vi "Calculate Distance to Target.vi"(10 "Diff Top X to Bottom X":dbl, 11 "Camera Height (pix)":dbl=320.0) -> (1 "Distance to Wall (in.)":dbl)   [LabVIEW 2019]
panel:
  in  "Camera Pix Hight Angle (degrees)":dbl=19.0
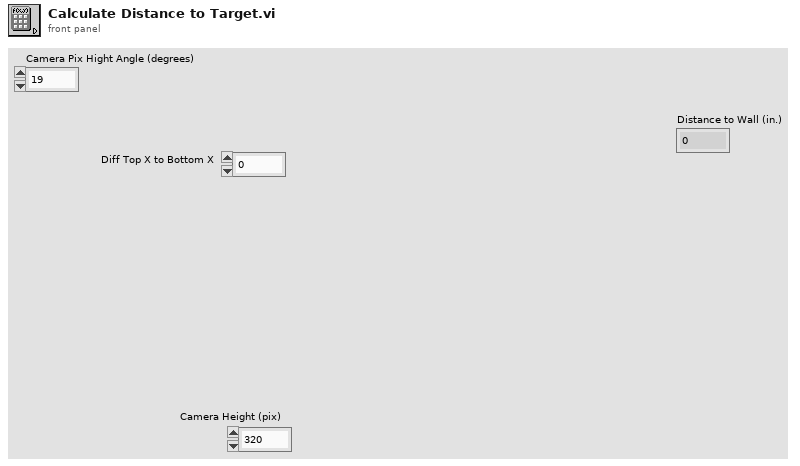
[diagram p1: front panel]
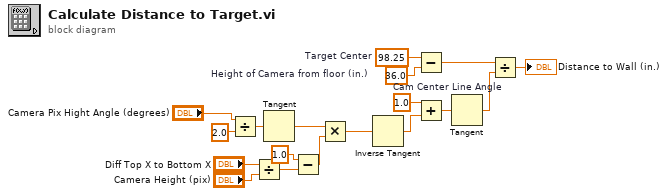
[diagram p0: block diagram]
diagram:
  w2 = 1.0  # Cam Center Line Angle
  w17 = 36.0  # Height of Camera from floor (in.)
  w18 = 98.25  # Target Center
  n1 = Divide(x="Camera Pix Hight Angle (degrees)", y=2.0) -> (x/y=w14:dbl)
  n2 = Divide(x="Diff Top X to Bottom X", y="Camera Height (pix)") -> (x/y=w3:dbl)
  n3 = Tangent(1:w14) -> (0:w12:dbl)
  n4 = Subtract(x=1.0, y=w3) -> (x-y=w11:dbl)
  n5 = Multiply(x=w12, y=w11) -> (x*y=w10:dbl)
  n6 = Inverse Tangent(1:w10) -> (0:w8:dbl)
  n7 = Subtract(x=w18, y=w17) -> (x-y=w16:dbl)
  n8 = Add(x=w2, y=w8) -> (x+y=w7:dbl)
  n9 = Tangent(1:w7) -> (0:w9:dbl)
  n10 = Divide(x=w16, y=w9) -> (x/y=→"Distance to Wall (in.)":dbl)
